vi "EnqueMessage.vi"(6 "timeout in ms (-1)":i32, 7 "Priority Message? (F)":bool, 8 "error in":errorcluster, 9 "Message Payload":variant, 10 "Message Command":string, 11 "Message que":T1) -> (0 "error out":errorcluster, 3 "Message que out":T1)   [LabVIEW 2018, in "MessageQue.lvlib"]
doc: "Transmit a message.\nFor a regular message, enqueue the message. For a priority message, enqueue it at the front of the queue.\n\nBolder Software LLC"
uses:
  MessageQue.lvlib
  MessageQue.ctl
  MessageCluster.ctl
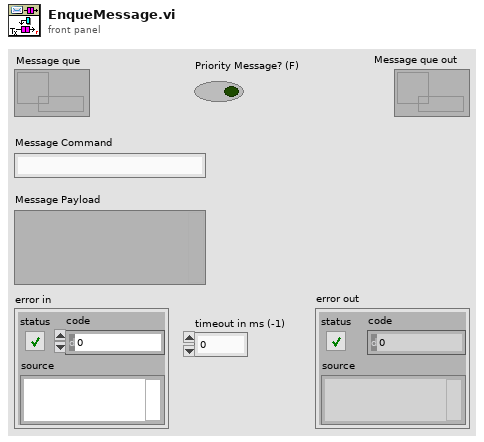
[diagram p1: front panel]
types:
  T1 = typedef "MessageQue.lvlib/MessageQue.ctl" = refnum<queue>
  T2 = typedef "MessageQue.lvlib/MessageCluster.ctl" = cluster{"Command":string, "Payload":variant}
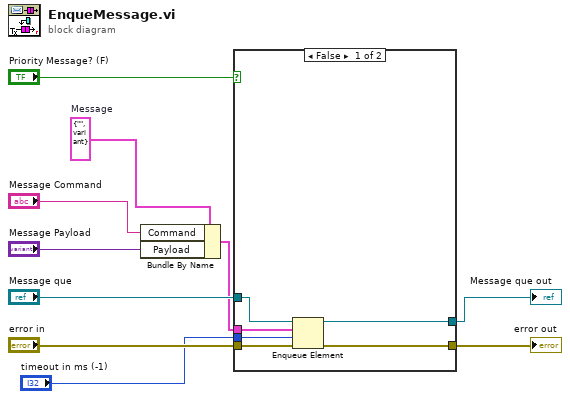
[diagram p0: block diagram]
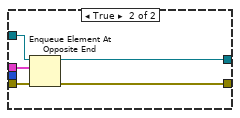
[diagram p2: hidden frame]
diagram:
  w10 = T2 {"Command"="", "Payload"=variant}  # Message
  n1 = Bundle By Name(cluster=w10, "Command"="Message Command", "Payload"="Message Payload") -> (w3:T2)
  n2 = case shown="False" "Priority Message? (F)" {
    tunnel: "error in" -> [w16 w21]
    tunnel: "Message que" -> [w15 w20]
    tunnel: w3 -> [w14 w19]
    tunnel: [w13 w17] -> w6
    tunnel: [w12 w18] -> w5
    tunnel: "timeout in ms (-1)" -> [w11 _]
    frame False {
      n3 = Enqueue Element(queue=w15, element=w14, timeout in ms (-1)=w11, error in (no error)=w16) -> (queue out=w12:T1, error out=w13:errorcluster)  [unwired: 1 out]
    }
    frame True {
      n4 = Enqueue Element At Opposite End(queue=w20, element=w19, error in (no error)=w21) -> (queue out=w18:T1, error out=w17:errorcluster)  [unwired: 1 in, 1 out]
    }
  }
  "error out" <- w6
  "Message que out" <- w5
